vi "03.2 Event-driven State Machine.vi"() -> ()   [LabVIEW 2019]
uses:
  03.2 States.ctl
  03.2 State Machine Data.ctl
  <vilib>/DAQmx/write.llb/DAQmx Write (Analog DBL 1Chan 1Samp).vi
  <vilib>/Utility/file.llb/Write Delimited Spreadsheet (string).vi
  <vilib>/Utility/file.llb/Write Delimited Spreadsheet (DBL).vi
  <vilib>/DAQmx/create/channels.llb/DAQmx Create Channel (AO-Voltage-Basic).vi
  <vilib>/DAQmx/miscellaneous.llb/DAQmx Fill In Error Info.vi
panel:
  in  "physical channels":tag
  in  "Threshold (RMS)":dbl
  in  "Generate Stimulus":bool
  in  "Stop":bool
  in  "Clear":bool
  in  "Acquire":bool
  out "Graph":dbl[][](graph)
  out "Thershold Exceeded?":bool
  out "RMS Result per Channel":dbl[](array[numeric])
  # "EVENTS"
  # "ANALYSIS"
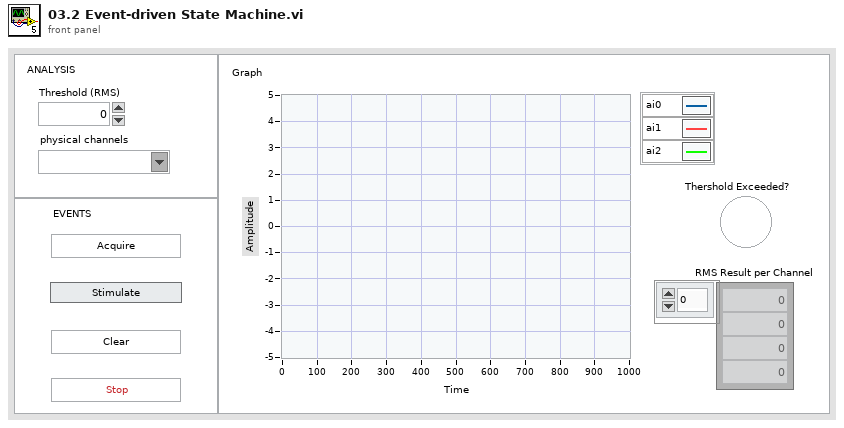
[diagram p1: front panel]
types:
  T1 = typedef "03.2 State Machine Data.ctl" = cluster{"Acquisition Data":dbl[][], "Stimulus?":bool}
  T2 = typedef "03.2 States.ctl" = enum16{"Initialize", "Update UI", "Update Stimulus", "Wait for event", "Acquire", "Analyze", "Log", "Clear", "Shutdown"}
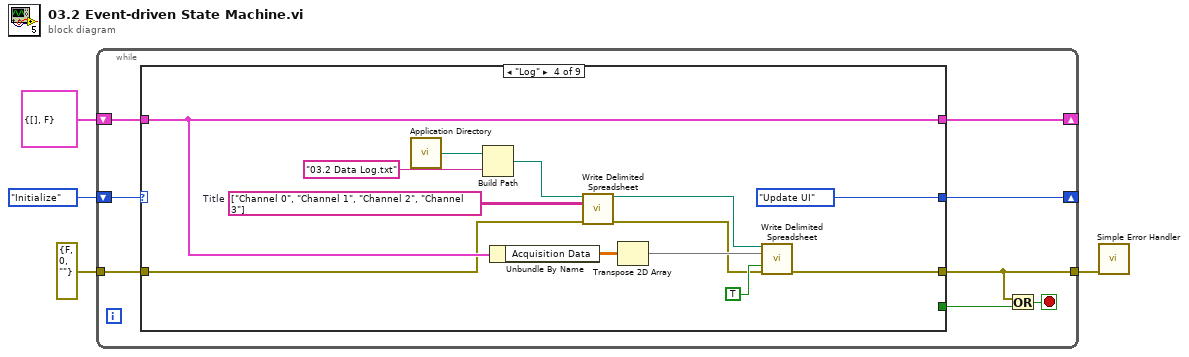
[diagram p0: block diagram]
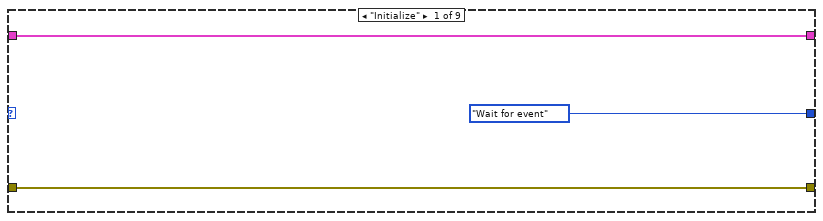
[diagram p2: hidden frame]
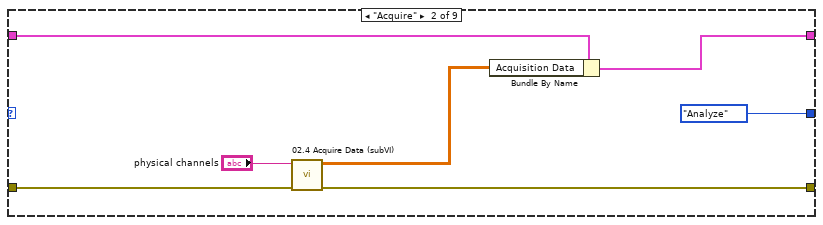
[diagram p3: hidden frame]
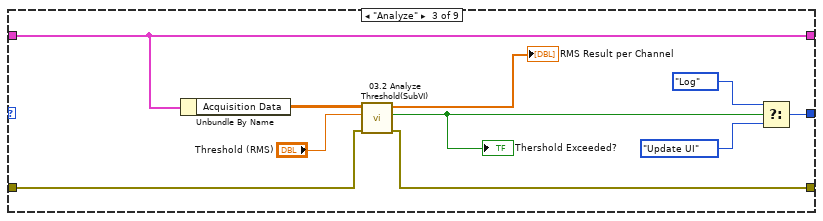
[diagram p4: hidden frame]
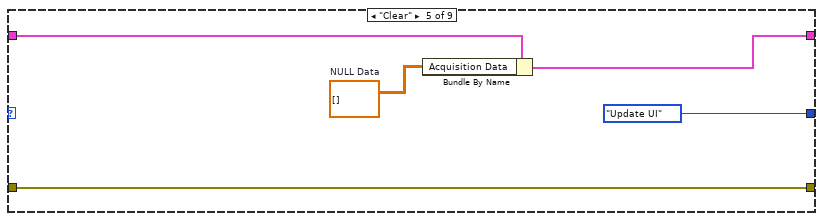
[diagram p5: hidden frame]
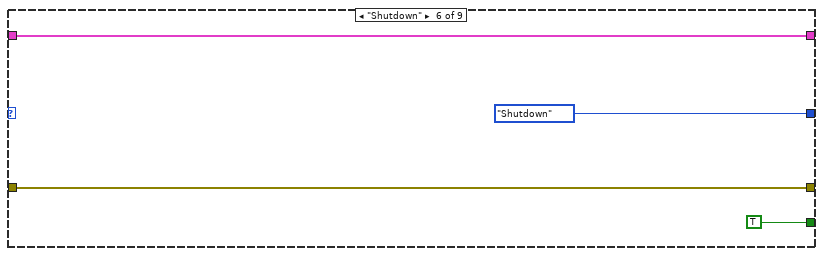
[diagram p6: hidden frame]
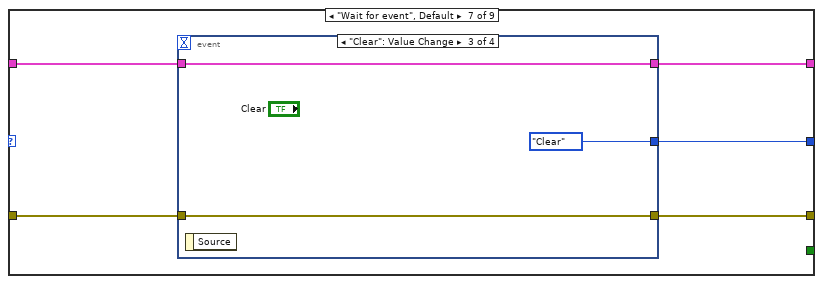
[diagram p7: hidden frame]
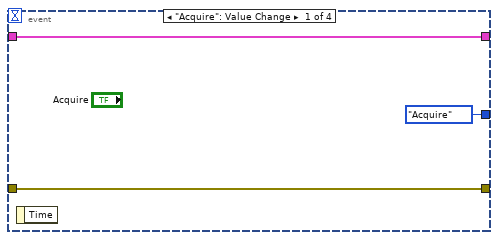
[diagram p8: hidden frame]
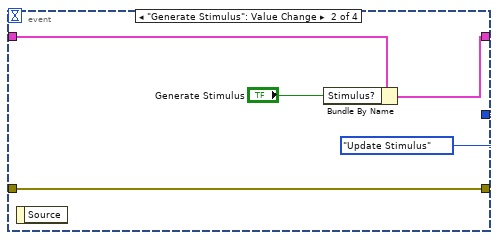
[diagram p9: hidden frame]
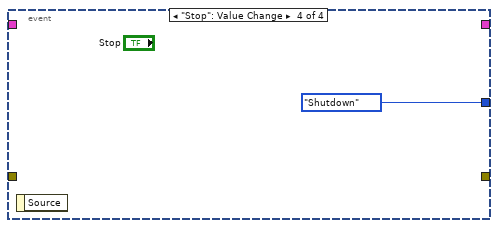
[diagram p10: hidden frame]
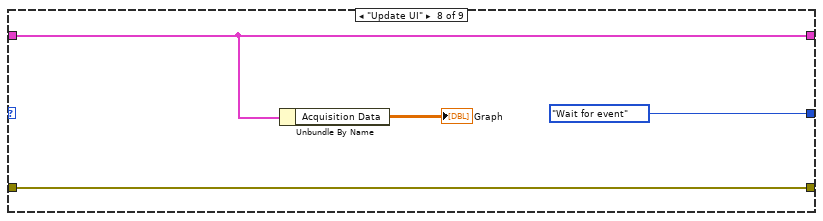
[diagram p11: hidden frame]
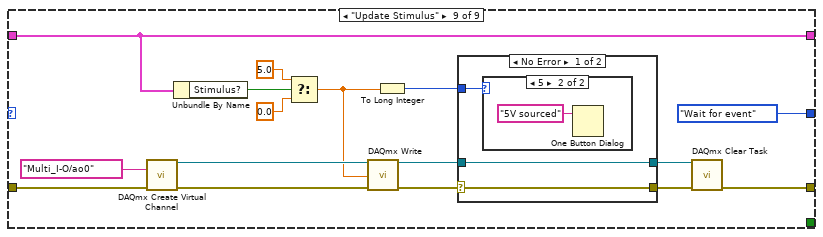
[diagram p12: hidden frame]
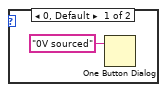
[diagram p13: hidden frame]
diagram:
  n1 = while {
    shift-right: [w11] -> _
    shift-left: 03.2_States."Initialize" ("State") -> [w12]
    tunnel: errorcluster {"status"=FALSE, "code"=0, "source"=""} ("error constant") -> [w10]
    tunnel: [w8] -> w2
    shift-right: [w7] -> _
    shift-left: T1 {"Acquisition Data"=[], "Stimulus?"=FALSE} -> [w6]
    stop <- w9 stop-if-true
    n2 = case shown="\"Log\"" w12 {
      tunnel: [03.2_States."Wait for event" ("State") 03.2_States."Analyze" ("State") w31 03.2_States."Update UI" ("State") 03.2_States."Update UI" ("State") 03.2_States."Shutdown" ("State") w59 03.2_States."Wait for event" ("State") 03.2_States."Wait for event" ("State")] -> w11
      tunnel: [w14 w18 w26 w43 w46 w52 w58 w73 w80] -> w8
      tunnel: w10 -> [w14 w19 w27 w33 w46 w52 w57 w73 w91]
      tunnel: [w15 w21 w25 w41 w49 w53 w56 w75 w77] -> w7
      tunnel: w6 -> [w15 w22 w25 w41 w50 w53 w55 w75 w77]
      tunnel: [_ _ _ _ _ TRUE _ _ _] -> w5
      frame "Initialize" {
      }
      frame "Acquire" {
        n3 = call "02.4 Acquire Data (subVI).vi"("Error In"=w19, "physical channels"="physical channels") -> ("error out"=w18:errorcluster, "2D DBL"=w20:dbl[][])  [unwired: 8 in]
        n4 = Bundle By Name(cluster=w22, "Acquisition Data"=w20) -> (w21:T1)
      }
      frame "Analyze" {
        n5 = Unbundle By Name(w25) -> ("Acquisition Data"=w32:dbl[][])
        n6 = call "03.2 Analyze Threshold(SubVI).vi"("Error In"=w27, "Threshold (RMS)"="Threshold (RMS)", "Data"=w32) -> ("Error Out"=w26:errorcluster, "Threshold exceeded?"=w28:bool, "RMS Results per Channel"=→"RMS Result per Channel":dbl[])  [unwired: 6 in]
        "Thershold Exceeded?" <- w28
        n7 = Select(t=03.2_States."Log" ("State"), s=w28, f=03.2_States."Update UI" ("State")) -> (s? t:f=w31:T2)
      }
      frame "Log" {
        w35 = string[][] [["Channel 0", "Channel 1", "Channel 2", "Channel 3"]]  # Title
        n8 = call <vilib>:"Application Directory.vi"() -> ("Application Directory"=w45:path)
        n9 = Build Path(base path=w45, name or relative path="03.2 Data Log.txt") -> (appended path=w36:path)
        n10 = Unbundle By Name(w41) -> ("Acquisition Data"=w40:dbl[][])
        n11 = call-poly <vilib>:"Write Delimited Spreadsheet.vi"("file path (dialog if empty)"=w36, "2D data"=w35, "error in (no error)"=w33) -> ("new file path (Not A Path if cancelled)"=w38:path, "error out"=w34:errorcluster)  [unwired: 11 in]
        n12 = Transpose 2D Array(2D array=w40) -> (transposed array=w39:dbl[][])
        n13 = call-poly <vilib>:"Write Delimited Spreadsheet.vi"("file path (dialog if empty)"=w38, "2D data"=w39, "append to file? (new file:F)"=TRUE, "error in (no error)"=w34) -> ("error out"=w43:errorcluster)  [unwired: 10 in, 1 out]
      }
      frame "Clear" {
        w48 = dbl[][] []  # NULL Data
        n14 = Bundle By Name(cluster=w50, "Acquisition Data"=w48) -> (w49:T1)
      }
      frame "Shutdown" {
      }
      frame "Wait for event", Default {
        n15 = event shown="[2] \"Clear\": Value Change" {
          selector: _ -> [_ _ _ _]
          dyn-events: _ -> [_ _ _ _]
          timeout: _ -> [_ _ _ _]
          tunnel: [03.2_States."Acquire" ("State") 03.2_States."Update Stimulus" ("State") 03.2_States."Clear" ("State") 03.2_States."Shutdown" ("State")] -> w59
          tunnel: [w61 w63 w68 _] -> w58
          tunnel: w57 -> [w61 w63 w68 _]
          tunnel: [w60 w65 w70 _] -> w56
          tunnel: w55 -> [w60 w67 w70 _]
          event "Acquire": Value Change {
            n16 = event-data() -> ()  [unwired: 1 in, 1 out]
          }
          event "Generate Stimulus": Value Change {
            n17 = event-data() -> ()  [unwired: 1 in, 1 out]
            n18 = Bundle By Name(cluster=w67, "Stimulus?"="Generate Stimulus") -> (w65:T1)
          }
          event "Clear": Value Change {
            n19 = event-data() -> ()  [unwired: 1 in, 1 out]
          }
          event "Stop": Value Change {
            n20 = event-data() -> ()  [unwired: 1 in, 1 out]
          }
        }
      }
      frame "Update UI" {
        n21 = Unbundle By Name(w75) -> ("Acquisition Data"=→"Graph":dbl[][])
      }
      frame "Update Stimulus" {
        n22 = call-poly <vilib>:"DAQmx Create Virtual Channel.vi"("physical channels"=tag "Multi_I-O/ao0", "error in"=w91) -> ("task out"=w89:refnum<k21>, "error out"=w90:errorcluster)  [unwired: 12 in]
        n23 = Unbundle By Name(w77) -> ("Stimulus?"=w88:bool)
        n24 = Select(t=5.0, s=w88, f=0.0) -> (s? t:f=w85:dbl)
        n25 = call-poly <vilib>:"DAQmx Write.vi"("task/channels in"=w89, "data"=w85, "error in"=w90) -> ("task out"=w83:refnum<k21>, "error out"=w84:errorcluster)  [unwired: 10 in, 1 out]
        n26 = To Long Integer(number=w85) -> (32bit integer=w78:i32)
        n27 = case shown="No Error" w84 {
          selector: w84 -> [w94 w97]
          tunnel: w83 -> [w93 w98]
          tunnel: [w94 w97] -> w82
          tunnel: [w93 w98] -> w81
          tunnel: w78 -> [w92 _]
          frame No Error {
            n28 = case shown="5" w92 {
              frame 0, Default {
                n29 = One Button Dialog(message="0V sourced") -> ()  [unwired: 1 in, 1 out]
              }
              frame 5 {
                n30 = One Button Dialog(message="5V sourced") -> ()  [unwired: 1 in, 1 out]
              }
            }
          }
          frame Error {
          }
        }
        n31 = call <vilib>:"DAQmx Clear Task.vi"("task in"=w81, "error in"=w82) -> ("error out"=w80:errorcluster)  [unwired: 13 in]
      }
    }
    n32 = Or(x=w8, y=w5) -> (x .or. y?=w9:bool)
  }
  n33 = call <vilib>:"Simple Error Handler.vi"("error in (no error)"=w2) -> ()  [unwired: 4 in, 5 out]
